vi "SavePupilCameraImage.vi"(5 "Save Format":enum16{"Png", "Raw"}(ring), 7 "Save Image?":bool, 8 "Block Folder":path, 9 "Subfolder":string="Eyetracker", 10 "Refnum in":T1) -> (2 "Refnum out (duplicate)":T1, 3 "ImageSaved":bool=TRUE)   [LabVIEW 2013]
uses:
  <vilib>/vision/Image Controls.llb/IMAQ Image.ctl
  <vilib>/Utility/file.llb/Write To Spreadsheet File (string).vi
  <vilib>/vision/NI_Vision_Development_Module.lvlib
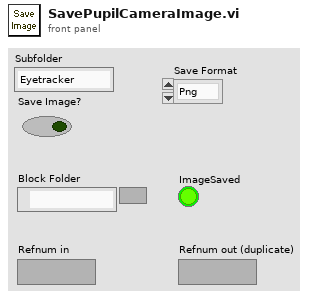
[diagram p1: front panel]
types:
  T1 = typedef "IMAQ Image.ctl" = refnum<image>
  T2 = enum16{"open", "replace", "create", "open or create", "replace or create", "replace or create with confirmation"}
  T3 = cluster{"Desired Font (Application)":enum16{"User-specified Font", "Application Font", "System Font", "Dialog Font"}, "[User-specified Font]":cluster{"Font Name":string, "Size":i16, "Strikeout?":bool, "Italic?":bool, "Underline?":bool, "Outline?":bool, "Shadow?":bool, "Bold?":bool, "Rotation Angle":dbl}, "Horizontal Alignment":i16, "Vertical Alignment":i16}
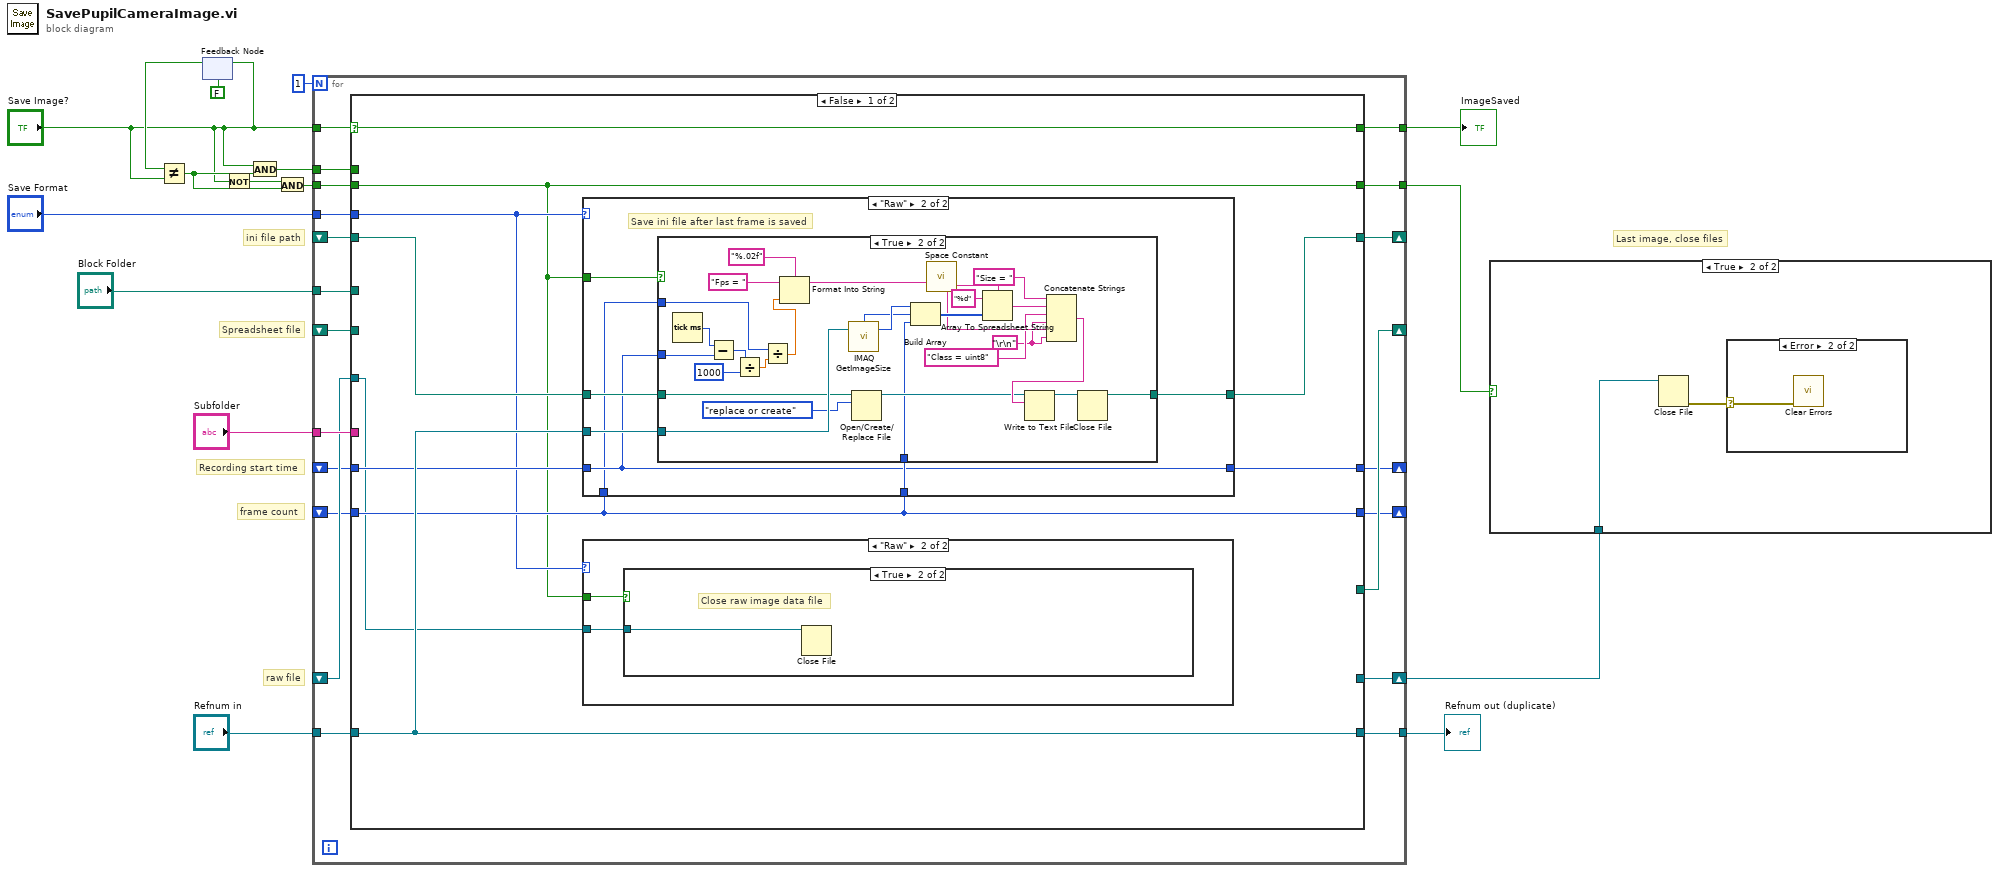
[diagram p0: block diagram]
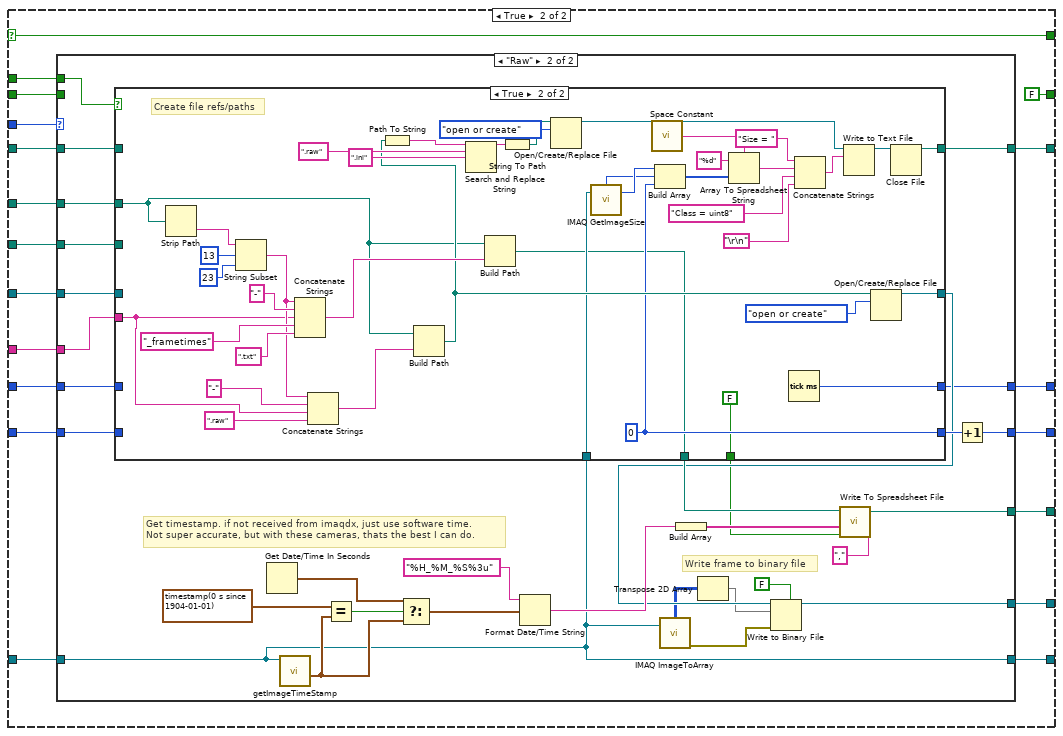
[diagram p8: hidden frame]
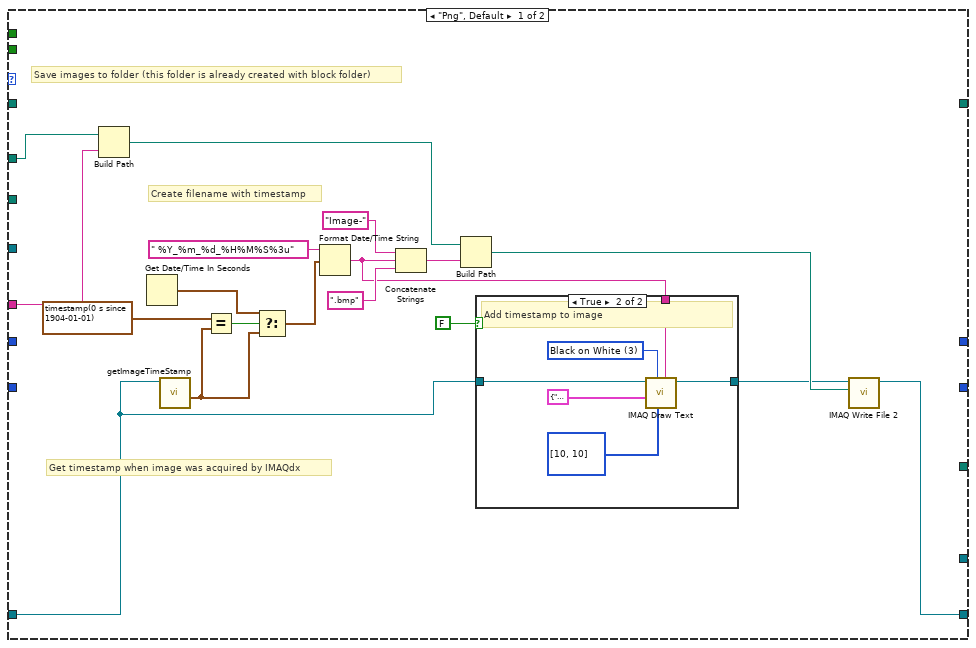
[diagram p9: hidden frame]
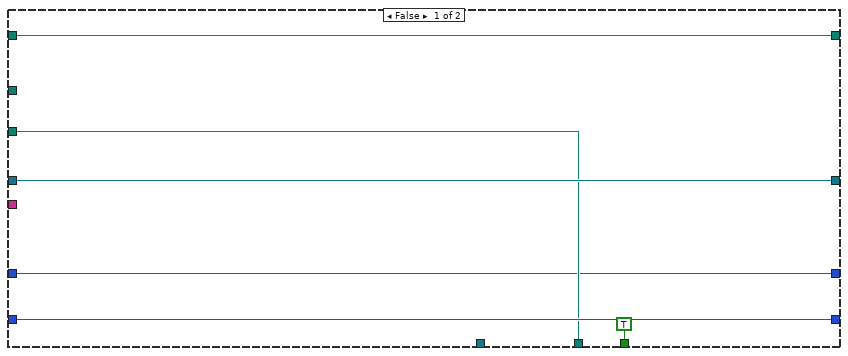
[diagram p11: hidden frame]
diagram:
  # "Recording start time"
  # "frame count"
  # "Spreadsheet file"
  # "raw file"
  # "ini file path"
  # "Last image, close files"
  n1 = feedback-in #1("Save Image?") -> ()
  n2 = feedback #1(FALSE ("Save Image?")) -> (w4:bool)
  n3 = Not Equal?(x=w4, y="Save Image?") -> (x != y?=w3:bool)
  n4 = Not(x="Save Image?") -> (.not. x?=w2:bool)
  n5 = And(x="Save Image?", y=w3) -> (x .and. y?=w6:bool)
  n6 = And(x=w2, y=w3) -> (x .and. y?=w5:bool)
  n7 = for {
    N: 1 -> [_]
    tunnel: [w36] -> w16
    tunnel: "Block Folder" -> [w35]
    tunnel: "Refnum in" -> [w34]
    tunnel: "Save Image?" -> [w33]
    tunnel: [w32] -> w10
    tunnel: "Subfolder" -> [w31]
    tunnel: "Save Format" -> [w30]
    tunnel: w6 -> [w29]
    shift-right: [w28] -> _
    shift-left: _ -> [w27]
    shift-right: [w26] -> w8
    shift-left: _ -> [w25]
    tunnel: w5 -> [w24]
    shift-right: [w23] -> _
    shift-left: _ -> [w22]
    tunnel: [w21] -> w9
    shift-right: [w20] -> _
    shift-left: _ -> [w19]
    shift-right: [w18] -> _
    shift-left: _ -> [w17]
    n8 = case shown="False" w33 {
      selector: w33 -> [w46 w102]
      tunnel: [w45 w104] -> w36
      tunnel: w35 -> [_ w105]
      tunnel: w34 -> [w45 w103]
      tunnel: [w46 w102] -> w32
      tunnel: w31 -> [_ w101]
      tunnel: w30 -> [w39 w100]
      tunnel: w29 -> [_ w99]
      tunnel: [_ w98] -> w26
      tunnel: [_ w97] -> w28
      tunnel: w27 -> [_ w96]
      tunnel: w25 -> [w37 w95]
      tunnel: w24 -> [w38 w94]
      tunnel: [w40 w93] -> w23
      tunnel: w22 -> [w40 w92]
      tunnel: [w38 FALSE ("Last Frame")] -> w21
      tunnel: [w43 w90] -> w20
      tunnel: w19 -> [w44 w89]
      tunnel: [w41 w88] -> w18
      tunnel: w17 -> [w42 w87]
      frame False {
        n9 = case shown="\"Raw\"" w39 {
          tunnel: w45 -> [_ w58]
          tunnel: w40 -> [_ w57]
          tunnel: w44 -> [w51 w56]
          tunnel: [w51 w55] -> w43
          tunnel: w38 -> [_ w54]
          tunnel: w42 -> [w50 w53]
          tunnel: [w50 w53] -> w41
          tunnel: w40 -> [_ w52]
          frame "Png", Default {
          }
          frame "Raw" {
            # "Save ini file after last frame is saved"
            n10 = case shown="True" w54 {
              tunnel: w58 -> [_ w78]
              tunnel: w57 -> [_ w76]
              tunnel: w56 -> [w59 w74]
              tunnel: [w59 w73] -> w55
              tunnel: w53 -> [_ w68]
              tunnel: w52 -> [_ w65]
              frame False {
              }
              frame True {
                w60 = "\r\n"
                n11 = Tick Count (ms)() -> (millisecond timer value=w69:u32)
                n12 = Subtract(x=w69, y=w68) -> (x-y=w67:u32)
                n13 = Divide(x=w67, y=u32 1000) -> (x/y=w64:dbl)
                n14 = Divide(x=w65, y=w64) -> (x/y=w63:dbl)
                n15 = Format Into String(format string="%.02f", initial string="Fps = ", w63) -> (resulting string=w62:string)  [unwired: 1 in, 1 out]
                n16 = call "IMAQ GetImageSize"("Image"=w78) -> ("Y Resolution"=w86:i32, "X Resolution"=w85:i32)  [unwired: 3 in, 1 out]
                n17 = Open/Create/Replace File(file path (use dialog)=w74, operation (0:open)=T2."replace or create") -> (refnum out=w77:refnum<file>)  [unwired: 4 in, 2 out]
                n18 = Build Array(w86, w85, w76) -> (w84:i32[])
                n19 = call <vilib>:"Space Constant.vi"() -> ("String"=w72:string)
                n20 = Array To Spreadsheet String(delimiter (Tab)=w72, array=w84, 3:"%d" ("format string")) -> (spreadsheet string=w82:string)
                n21 = Concatenate Strings("Size = " ("string"), w82, "Class = uint8" ("string"), w60, w62, w60) -> (w79:string)
                n22 = Write to Text File(file (use dialog)=w77, text=w79) -> (refnum out=w80:refnum<file>)  [unwired: 2 in, 2 out]
                n23 = Close File(refnum=w80) -> (path=w73:path)  [unwired: 1 in, 1 out]
              }
            }
          }
        }
        n24 = case shown="\"Raw\"" w39 {
          tunnel: w38 -> [_ w48]
          tunnel: w37 -> [_ w47]
          frame "Png", Default {
          }
          frame "Raw" {
            n25 = case shown="True" w48 {
              tunnel: w47 -> [_ w49]
              frame False {
              }
              frame True {
                # "Close raw image data file"
                n26 = Close File(refnum=w49) -> ()  [unwired: 1 in, 2 out]
              }
            }
          }
        }
      }
      frame True {
        n27 = case shown="\"Raw\"" w100 {
          tunnel: w105 -> [w118 w148]
          tunnel: [w115 w135] -> w104
          tunnel: w103 -> [w113 w135]
          tunnel: w101 -> [w111 w149]
          tunnel: w99 -> [_ w142]
          tunnel: [_ w150] -> w98
          tunnel: [_ w147] -> w97
          tunnel: w96 -> [_ w146]
          tunnel: w95 -> [_ w145]
          tunnel: w94 -> [_ _]
          tunnel: [_ w143] -> w93
          tunnel: w92 -> [_ w144]
          tunnel: [_ w140] -> w90
          tunnel: w89 -> [_ w138]
          tunnel: [_ w134] -> w88
          tunnel: w87 -> [_ w133]
          frame "Png", Default {
            # "Get timestamp when image was acquired by IMAQdx"
            # "Save images to folder (this folder is already created with block folder)"
            # "Create filename with timestamp"
            n28 = Build Path(base path=w118, name or relative path=w111) -> (appended path=w117:path)
            n29 = Get Date/Time In Seconds() -> (seconds since 1Jan1904=w109:timestamp)
            n30 = call "getImageTimeStamp.vi"("Image refnum in"=w113) -> ("System Time Stamp"=w108:timestamp)  [unwired: 9 in, 1 out]
            n31 = Equal?(x=timestamp(0 s since 1904-01-01), y=w108) -> (x = y?=w110:bool)
            n32 = Select(t=w109, s=w110, f=w108) -> (s? t:f=w107:timestamp)
            n33 = Format Date/Time String(time format string (%c)=" %Y_%m_%d_%H%M%S%3u", seconds (now)=w107) -> (date/time string=w116:string)  [unwired: 1 in]
            n34 = Concatenate Strings("Image-" ("string"), w116, ".bmp" ("string")) -> (w122:string)
            n35 = Build Path(base path=w117, name or relative path=w122) -> (appended path=w123:path)
            n36 = case shown="True" FALSE {
              tunnel: w116 -> [_ w130]
              tunnel: w113 -> [w124 w126]
              tunnel: [w124 w125] -> w112
              frame False {
              }
              frame True {
                w127 = 3 items=["White", "Black", "Inverted", "Black on White", "White on Black"] ("Color")
                # "Add timestamp to image"
                n37 = call "IMAQ Draw Text"("String"=w130, "Insertion Point"=i32[] [10, 10], "Color"=w127, "Font, Size & Style"=T3 {"Desired Font (Application)"=enum."User-specified Font", "[User-specified Font]"={"Font Name"="", "Size"=26, "Strikeout?"=FALSE, "Italic?"=FALSE, "Underline?"=FALSE, "Outline?"=FALSE, "Shadow?"=FALSE, "Bold?"=FALSE, "Rotation Angle"=0.0}, "Horizontal Alignment"=0, "Vertical Alignment"=1}, "Image Src"=w126) -> ("Image Dst Out"=w125:T1)  [unwired: 3 in, 3 out]
              }
            }
            n38 = call-poly "IMAQ Write File 2"("File Path"=w123, "Image"=w112) -> ("Image Out (duplicate)"=w115:T1)  [unwired: 8 in, 1 out]
          }
          frame "Raw" {
            # "Write frame to binary file"
            # "Get timestamp. if not received from imaqdx, just use software time. \nNot super accurate, but with these cameras, thats the best I can do."
            n39 = case shown="True" w142 {
              tunnel: w149 -> [_ w194]
              tunnel: w148 -> [_ w173]
              tunnel: w146 -> [w165 _]
              tunnel: [w167 w195] -> w137
              tunnel: w145 -> [w167 _]
              tunnel: [w166 w175] -> w141
              tunnel: w144 -> [w166 _]
              tunnel: [w164 w178] -> w140
              tunnel: w135 -> [_ w176]
              tunnel: [w165 w174] -> w139
              tunnel: w138 -> [w164 _]
              tunnel: [TRUE FALSE] -> w136
              tunnel: [w162 w168] -> w134
              tunnel: w133 -> [w162 _]
              frame False {
              }
              frame True {
                w175 = 0
                # "Create file refs/paths"
                n40 = Strip Path(path=w173) -> (name=w203:string)  [unwired: 1 out]
                n41 = String Subset(string=w203, offset (0)=13, length (rest)=23 ("length (rest)")) -> (substring=w198:string)
                n42 = Concatenate Strings(w198, "-" ("string"), w194, "_frametimes" ("string"), ".txt" ("string")) -> (w207:string)
                n43 = Concatenate Strings(w198, "-" ("string"), w194, ".raw" ("string")) -> (w197:string)
                n44 = Build Path(base path=w173, name or relative path=w197) -> (appended path=w189:path)
                n45 = Path To String(path=w189) -> (string=w190:string)
                n46 = Search and Replace String(input string=w190, search string=".raw", replace string=".ini" ("replace string (\"\")")) -> (result string=w193:string)  [unwired: 5 in, 3 out]
                n47 = Build Path(base path=w173, name or relative path=w207) -> (appended path=w174:path)
                n48 = String To Path(string=w193) -> (path=w188:path)
                n49 = Open/Create/Replace File(file path (use dialog)=w188, operation (0:open)=T2."open or create") -> (refnum out=w177:refnum<file>)  [unwired: 4 in, 2 out]
                n50 = call "IMAQ GetImageSize"("Image"=w176) -> ("Y Resolution"=w186:i32, "X Resolution"=w185:i32)  [unwired: 3 in, 1 out]
                n51 = call <vilib>:"Space Constant.vi"() -> ("String"=w171:string)
                n52 = Build Array(w186, w185, w175) -> (w184:i32[])
                n53 = Array To Spreadsheet String(delimiter (Tab)=w171, array=w184, 3:"%d" ("format string")) -> (spreadsheet string=w182:string)
                n54 = Tick Count (ms)() -> (millisecond timer value=w168:u32)
                n55 = Concatenate Strings("Size = " ("string"), w182, "Class = uint8" ("string"), "\r\n") -> (w179:string)
                n56 = Write to Text File(file (use dialog)=w177, text=w179) -> (refnum out=w180:refnum<file>)  [unwired: 2 in, 2 out]
                n57 = Open/Create/Replace File(file path (use dialog)=w189, operation (0:open)=T2."open or create") -> (refnum out=w195:refnum<file>)  [unwired: 4 in, 2 out]
                n58 = Close File(refnum=w180) -> (path=w178:path)  [unwired: 1 in, 1 out]
              }
            }
            n59 = Get Date/Time In Seconds() -> (seconds since 1Jan1904=w159:timestamp)
            n60 = call "getImageTimeStamp.vi"("Image refnum in"=w135) -> ("System Time Stamp"=w156:timestamp)  [unwired: 9 in, 1 out]
            n61 = Equal?(x=timestamp(0 s since 1904-01-01), y=w156) -> (x = y?=w160:bool)
            n62 = Select(t=w159, s=w160, f=w156) -> (s? t:f=w158:timestamp)
            n63 = Format Date/Time String(time format string (%c)="%H_%M_%S%3u", seconds (now)=w158) -> (date/time string=w152:string)  [unwired: 1 in]
            n64 = call "IMAQ ImageToArray"("Image"=w135) -> ("error out"=w154:errorcluster, "Image Pixels (U8)"=w132:u8[][])  [unwired: 3 in, 3 out]
            n65 = Build Array(w152) -> (w151:string[])
            n66 = Transpose 2D Array(2D array=w132) -> (transposed array=w131:u8[][])
            n67 = Write to Binary File(file (use dialog)=w137, data=w131, error in=w154, 5:FALSE ("prepend array or string size? (T)")) -> (refnum out=w150:refnum<file>)  [unwired: 2 in, 2 out]
            n68 = call-poly <vilib>:"Write To Spreadsheet File.vi"("delimiter (\\t)"="," ("delimiter (\\t)"), "append to file? (new file:F)"=w136, "1D data"=w151, "file path (dialog if empty)"=w139) -> ("new file path (Not A Path if cancelled)"=w147:path)  [unwired: 3 in, 1 out]
            n69 = Increment(x=w141) -> (x+1=w143:i32)
          }
        }
      }
    }
  }
  "Refnum out (duplicate)" <- w16
  "ImageSaved" <- w10
  n70 = case shown="True" w9 {
    tunnel: w8 -> [_ w209]
    frame False {
    }
    frame True {
      n71 = Close File(refnum=w209) -> (error out=w208:errorcluster)  [unwired: 1 in, 1 out]
      n72 = case shown="Error" w208 {
        selector: w208 -> [_ w210]
        frame No Error {
        }
        frame Error {
          n73 = call <vilib>:"Clear Errors.vi"("error in (no error)"=w210) -> ()  [unwired: 6 in, 1 out]
        }
      }
    }
  }
